vi "HEWH Search Tmax1 Location.vi"(8 "error in (no error)":errorcluster, 10 "Non-Draw/Draw Index":i32[][](array[numeric]), 11 "Tmax1 Index":i32) -> (0 "error out":errorcluster, 1 "Tmax1 Occurred During Draw":bool, 2 "Tmax1 Recovery Draw #":i32, 3 "Condition Found?":bool[](array[boolean]))   [LabVIEW 2023]
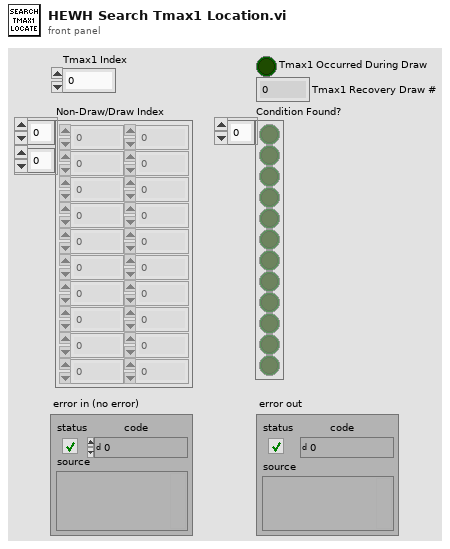
[diagram p1: front panel]
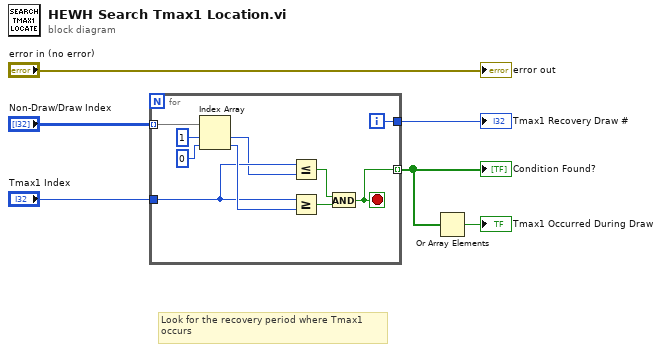
[diagram p0: block diagram]
diagram:
  # "Look for the recovery period where Tmax1 \noccurs"
  n1 = for {
    tunnel: "Tmax1 Index" -> [w8]
    tunnel: "Non-Draw/Draw Index" -> [w15] mode=indexing
    tunnel: [w16] -> w5
    tunnel: [w9] -> w2 mode=indexing
    i -> [w16]
    stop <- w9 stop-if-true
    n2 = Index Array(array=w15, index #1=1 ("index"), index #2=0 ("index")) -> (element #1=w7:i32, element #2=w12:i32)
    n3 = Less Or Equal?(x=w8, y=w7) -> (x <= y?=w11:bool)
    n4 = Greater Or Equal?(x=w8, y=w12) -> (x >= y?=w10:bool)
    n5 = And(x=w11, y=w10) -> (x .and. y?=w9:bool)
  }
  "Condition Found?" <- w2
  "Tmax1 Recovery Draw #" <- w5
  n6 = Or Array Elements(Boolean array=w2) -> (logical OR=→"Tmax1 Occurred During Draw":bool)
  "error out" <- "error in (no error)"
